vi "sequence_tick.vi"() -> ()   [LabVIEW 2018]
panel:
  out "x-y":u32
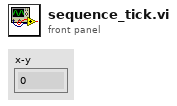
[diagram p1: front panel]
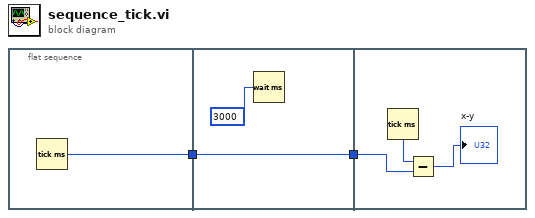
[diagram p0: block diagram]
diagram:
  n1 = flat-sequence {
    tunnel: [w3] -> w1
    tunnel: [w4] -> w2
    tunnel: w1 -> [w4]
    tunnel: w2 -> [w7]
    frame #0 {
      n2 = Tick Count (ms)() -> (millisecond timer value=w3:u32)
    }
    frame #1 {
      n3 = Wait (ms)(milliseconds to wait=u32 3000 ("대기 시간 (ms)")) -> ()  [unwired: 1 out]
    }
    frame #2 {
      n4 = Tick Count (ms)() -> (millisecond timer value=w8:u32)
      n5 = Subtract(x=w8, y=w7) -> (x-y=→"x-y":u32)
    }
  }
